vi "Register Broadcast.vi"() -> ()   [LabVIEW 2020, in "TCPRouter ClientAPI Examples.lvlib"]
uses:
  _addons/TCP-Router/ClientAPI/Def-TCP-Router Status Data.ctl
  b3b63605-1016-4be4-a788-12e3256b011c.vi
  TCPRouter ClientAPI Examples.lvlib
  _addons/TCP-Router/ClientAPI/TcpRouter-Client.lvclass
panel:
  out "# elements in queue":i32
  out "current time":timestamp
  out "element":T1
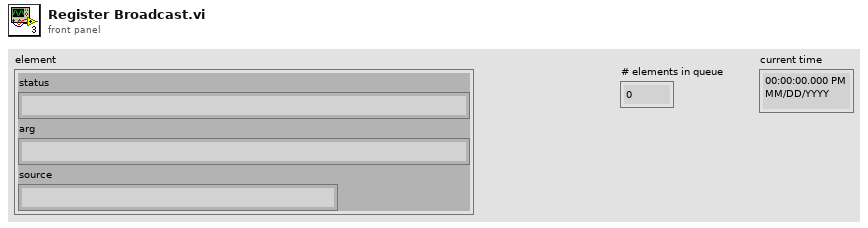
[diagram p1: front panel]
types:
  T1 = typedef "CSM-TCP-Router.lvlib/TcpRouter-Client.lvclass/Def-TCP-Router Status Data.ctl" = cluster{"status":string, "arg":string, "source":string}
  T2 = cluster{"IP Address":string, "Port":u16, "ConnectTMO":i32}
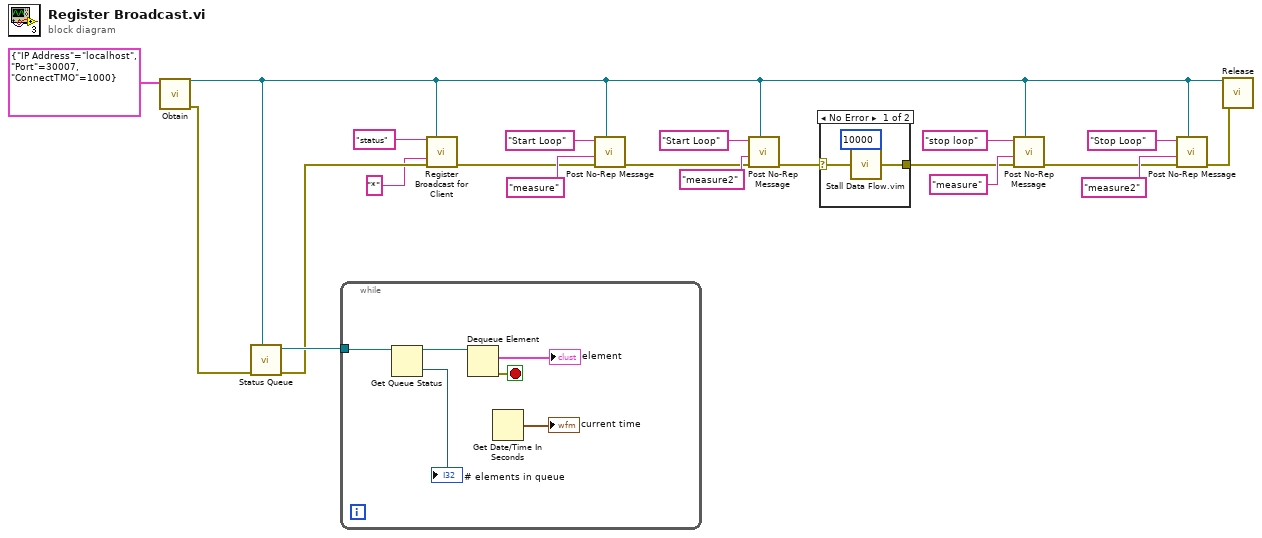
[diagram p0: block diagram]
diagram:
  n1 = call "Obtain.vi"("Connection"=T2 {"IP Address"="localhost", "Port"=30007, "ConnectTMO"=1000}) -> ("error out"=w13:errorcluster, "TcpRouter-Client out"=w1:refnum<class "TcpRouter-Client.lvclass">)  [unwired: 9 in]
  n2 = call "Status Queue.vi"("TcpRouter-Client in"=w1, "error in (no error)"=w13) -> ("error out"=w12:errorcluster, "StatusQueue"=w15:refnum<queue>)  [unwired: 8 in]
  n3 = while {
    tunnel: w15 -> [w27]
    stop <- w26 stop-if-true
    n4 = Get Queue Status(queue=w27) -> (queue out=w23:refnum<queue>, # elements in queue=→"# elements in queue":i32)  [unwired: 2 in, 6 out]
    n5 = Dequeue Element(queue=w23) -> (element=→"element":T1, error out=w26:errorcluster)  [unwired: 2 in, 2 out]
    n6 = Get Date/Time In Seconds() -> (seconds since 1Jan1904=→"current time":timestamp)
  }
  n7 = call "Register Broadcast for Client.vi"("Status"="status" ("CSM Name"), "TcpRouter-Client in"=w1, "CSM Name"="*" ("Source CSM Name (* as Default)"), "error in (no error)"=w12) -> ("error out"=w14:errorcluster)  [unwired: 10 in, 1 out]
  n8 = call "Post No-Rep Message.vi"("TcpRouter-Client in"=w1, "error in (no error)"=w14, "Target Module"="measure", "State"="Start Loop") -> ("error out"=w7:errorcluster)  [unwired: 7 in]
  n9 = call "Post No-Rep Message.vi"("TcpRouter-Client in"=w1, "error in (no error)"=w7, "Target Module"="measure2", "State"="Start Loop") -> ("error out"=w6:errorcluster)  [unwired: 7 in]
  n10 = case shown="No Error" w6 {
    selector: w6 -> [w28 w31]
    tunnel: [w30 w31] -> w16
    frame No Error {
      n11 = call "Stall Data Flow.vim"("value in"=w28, "milliseconds to wait"=u32 10000) -> ("value out"=w30:errorcluster)  [unwired: 1 out]
    }
    frame Error {
    }
  }
  n12 = call "Post No-Rep Message.vi"("TcpRouter-Client in"=w1, "error in (no error)"=w16, "Target Module"="measure", "State"="stop loop") -> ("error out"=w3:errorcluster)  [unwired: 7 in]
  n13 = call "Post No-Rep Message.vi"("TcpRouter-Client in"=w1, "error in (no error)"=w3, "Target Module"="measure2", "State"="Stop Loop") -> ("error out"=w2:errorcluster)  [unwired: 7 in]
  n14 = call "Release.vi"("error in (no error)"=w2, "TcpRouter-Client in"=w1) -> ()  [unwired: 9 in, 1 out]
